vi "Range (2D).vi"(1 "Array":dbl[][](array[numeric])) -> (0 "Range":dbl[](array[numeric]))   [LabVIEW 2020]
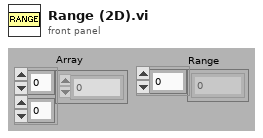
[diagram p1: front panel]
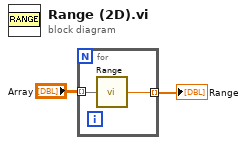
[diagram p0: block diagram]
diagram:
  n1 = for {
    tunnel: "Array" -> [w4] mode=indexing
    tunnel: [w3] -> w1 mode=indexing
    n2 = call "Range.vi"("Array"=w4) -> ("Range"=w3:dbl)
  }
  "Range" <- w1
